vi "fahrenheit2celsius.vi"() -> ()   [LabVIEW 2017]
panel:
  out "Thermometer":dbl(slide) scale=-20.0..130.0
  in  "Farenheit":dbl(slide) scale=-10.0..220.0
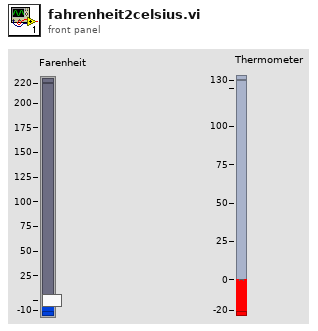
[diagram p1: front panel]
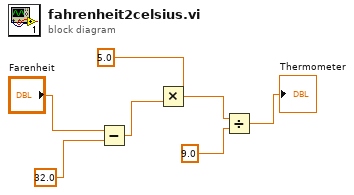
[diagram p0: block diagram]
diagram:
  n1 = Subtract(x="Farenheit", y=32.0) -> (x-y=w5:dbl)
  n2 = Multiply(x=5.0, y=w5) -> (x*y=w2:dbl)
  n3 = Divide(x=w2, y=9.0) -> (x/y=→"Thermometer":dbl)
